vi "RobotSimulator.vi"() -> ()   [LabVIEW 2018]
uses:
  Robot-Project/Drive/Implementation/Drive Setpoints.ctl
  Robot-Project/Drive/Implementation/Drive Operations.ctl
  Controls/PurePursuit/RobotNeededPathData.ctl
  Robot-Project/Drive/DriveState.ctl
  <extravilib>/ChannelInstances/Lossy Stream-c(dbl,dbl,dbl,c(dbl,dbl))/Write With Abort.vi
  <extravilib>/ChannelInstances/Lossy Stream-c(dbl,dbl,dbl,c(dbl,dbl))/Read With Abort.vi
  <extravilib>/ChannelInstances/Lossy Stream-c(dbl,dbl,dbl,c(dbl,dbl))/Endpoint.vi
  <extravilib>/ChannelInstances/Lossy Stream-c(dbl,dbl,dbl,c(dbl,dbl))/EndpointRead.vi
  Robot-Project/Drive/Implementation/Drive Published Globals.vi
  <extravilib>/ChannelInstances/Lossy Stream-c(dbl,dbl,dbl,c(dbl,dbl))/Instantiate.vi
  <extravilib>/ChannelInstances/Lossy Stream-c(dbl,dbl,dbl,c(dbl,dbl))/)Channel.vi
  <resource>/ChannelSupport/_ChannelSupport/WaitIfNeeded.vi
  <vilib>/addons/control/pid/pid.llb/PID (DBL).vi
  Robot-Project/Configuration/Constants.vi
  <vilib>/addons/control/pid/NI_PID_pid.lvlib
  <extravilib>/ChannelInstances/Lossy Stream-c(dbl,dbl,dbl,c(dbl,dbl)).lvlib
panel:
  in  "Path":cluster{dbl, dbl}[](array[cluster])
  in  "Angle Addition":dbl(slide) scale=-180.0..180.0
  in  "Target":cluster{dbl, dbl}={200.0, 200.0}
  out "Current\nCmd":string="Started at  14:51:47.884\nDefault: Reserve,  L 0.0, R 0.0, D 0.000000"
  in  "Go":bool
  out "Loop Iterations":i32
  in  "Gains 2":T1={"Gains"={"FFV"=0.0055, "FFA"=0.0025, "Vel PID"={"P"=0.05, "I"=0.0, "D"=0.0}}, "Pos PID"={"P"=0.05, "I"=0.0, "D"=0.0}, "MinVoltage"=0.0, "Effective Trackwidth"=29.0, "Effective Trackwidth CCW"=29.0} {"Pos PID"."D" format="%.3f"; "Pos PID"."I" format="%.3f"; "Pos PID"."P" format="%.3f"; "Gains"."Vel PID"."D" format="%.3f"; "Gains"."Vel PID"."I" format="%.3f"; "Gains"."Vel PID"."P" format="%.3f"}
  out "Graph":cluster{cluster{"x":dbl, "y":dbl}[]}[](graph)=[{[]}, {[{"x"=19.5, "y"=127.60329985652797}, {"x"=31.499289530461766, "y"=127.73387843115106}]}, {[{"x"=0.0, "y"=0.0}]}, {[{"x"=19.5, "y"=127.60329985652797}, {"x"=19.5, "y"=127.60329985652797}, {"x"=19.5, "y"=127.60329985652797}, {"x"=19.5, "y"=127.60329985652797}, {"x"=19.5, "y"=127.60329985652797}, {"x"=19.5, "y"=127.60329985652797}, {"x"=19.5, "y"=127.60329985652797}, {"x"=19.5, "y"=127.60329985652797}, {"x"=19.5, "y"=127.60329985652797}, {"x"=19.5, "y"=127.60329985652797}, {"x"=19.5, "y"=127.60329985652797}, {"x"=19.5, "y"=127.60329985652797}, {"x"=19.5, "y"=127.60329985652797}, {"x"=19.5, "y"=127.60329985652797}, {"x"=19.5, "y"=127.60329985652797}, {"x"=19.5, "y"=127.60329985652797}, {"x"=19.5, "y"=127.60329985652797}, {"x"=19.5, "y"=127.60329985652797}, {"x"=19.5, "y"=127.60329985652797}, {"x"=19.5, "y"=127.60329985652797}, {"x"=19.5, "y"=127.60329985652797}, {"x"=19.5, "y"=127.60329985652797}, {"x"=19.5, "y"=127.60329985652797}, {"x"=19.5, "y"=127.60329985652797}, {"x"=19.5, "y"=127.60329985652797}, {"x"=19.5, "y"=127.60329985652797}, {"x"=19.5, "y"=127.60329985652797}, {"x"=19.5, "y"=127.60329985652797}, {"x"=19.5, "y"=127.60329985652797}, {"x"=19.5, "y"=127.60329985652797}, {"x"=19.5, "y"=127.60329985652797}]}, {[{"x"=inf, "y"=nan}, {"x"=inf, "y"=nan}, {"x"=inf, "y"=nan}, {"x"=inf, "y"=nan}, {"x"=inf, "y"=nan}, {"x"=inf, "y"=nan}, {"x"=inf, "y"=nan}, {"x"=inf, "y"=nan}, {"x"=nan, "y"=nan}, {"x"=nan, "y"=nan}, {"x"=nan, "y"=nan}, {"x"=nan, "y"=nan}, {"x"=nan, "y"=nan}, {"x"=nan, "y"=nan}, {"x"=nan, "y"=nan}, {"x"=nan, "y"=nan}, {"x"=nan, "y"=-inf}, {"x"=nan, "y"=-inf}, {"x"=nan, "y"=-inf}, {"x"=nan, "y"=-inf}, {"x"=nan, "y"=-inf}, {"x"=nan, "y"=-inf}, {"x"=nan, "y"=-inf}, {"x"=inf, "y"=-inf}, {"x"=inf, "y"=-inf}, {"x"=inf, "y"=-inf}, {"x"=inf, "y"=-inf}, {"x"=inf, "y"=-inf}, {"x"=inf, "y"=-inf}, {"x"=inf, "y"=-inf}, {"x"=inf, "y"=-inf}]}]
  out "Right Output":dbl
  out "Left Output":dbl
  in  "Config":T2={"Gear Reduction"=8.7, "Wheel Radius (m)"=0.076, "# Motors"=3, "coeff of friction"=0.1, "Mass (kg)"=55.0, "Motor"={"Ke (V)"=0.0183, "R (ohms)"=0.14, "KT (Nm/A)"=0.0183, "Tf (Nm)"=0.015}}
  in  "Position":dbl=3.0
  in  "Gains":T3={"FFV"=0.0059, "FFA"=0.0019, "Vel PID"={"P"=0.01, "I"=0.0, "D"=0.0}}
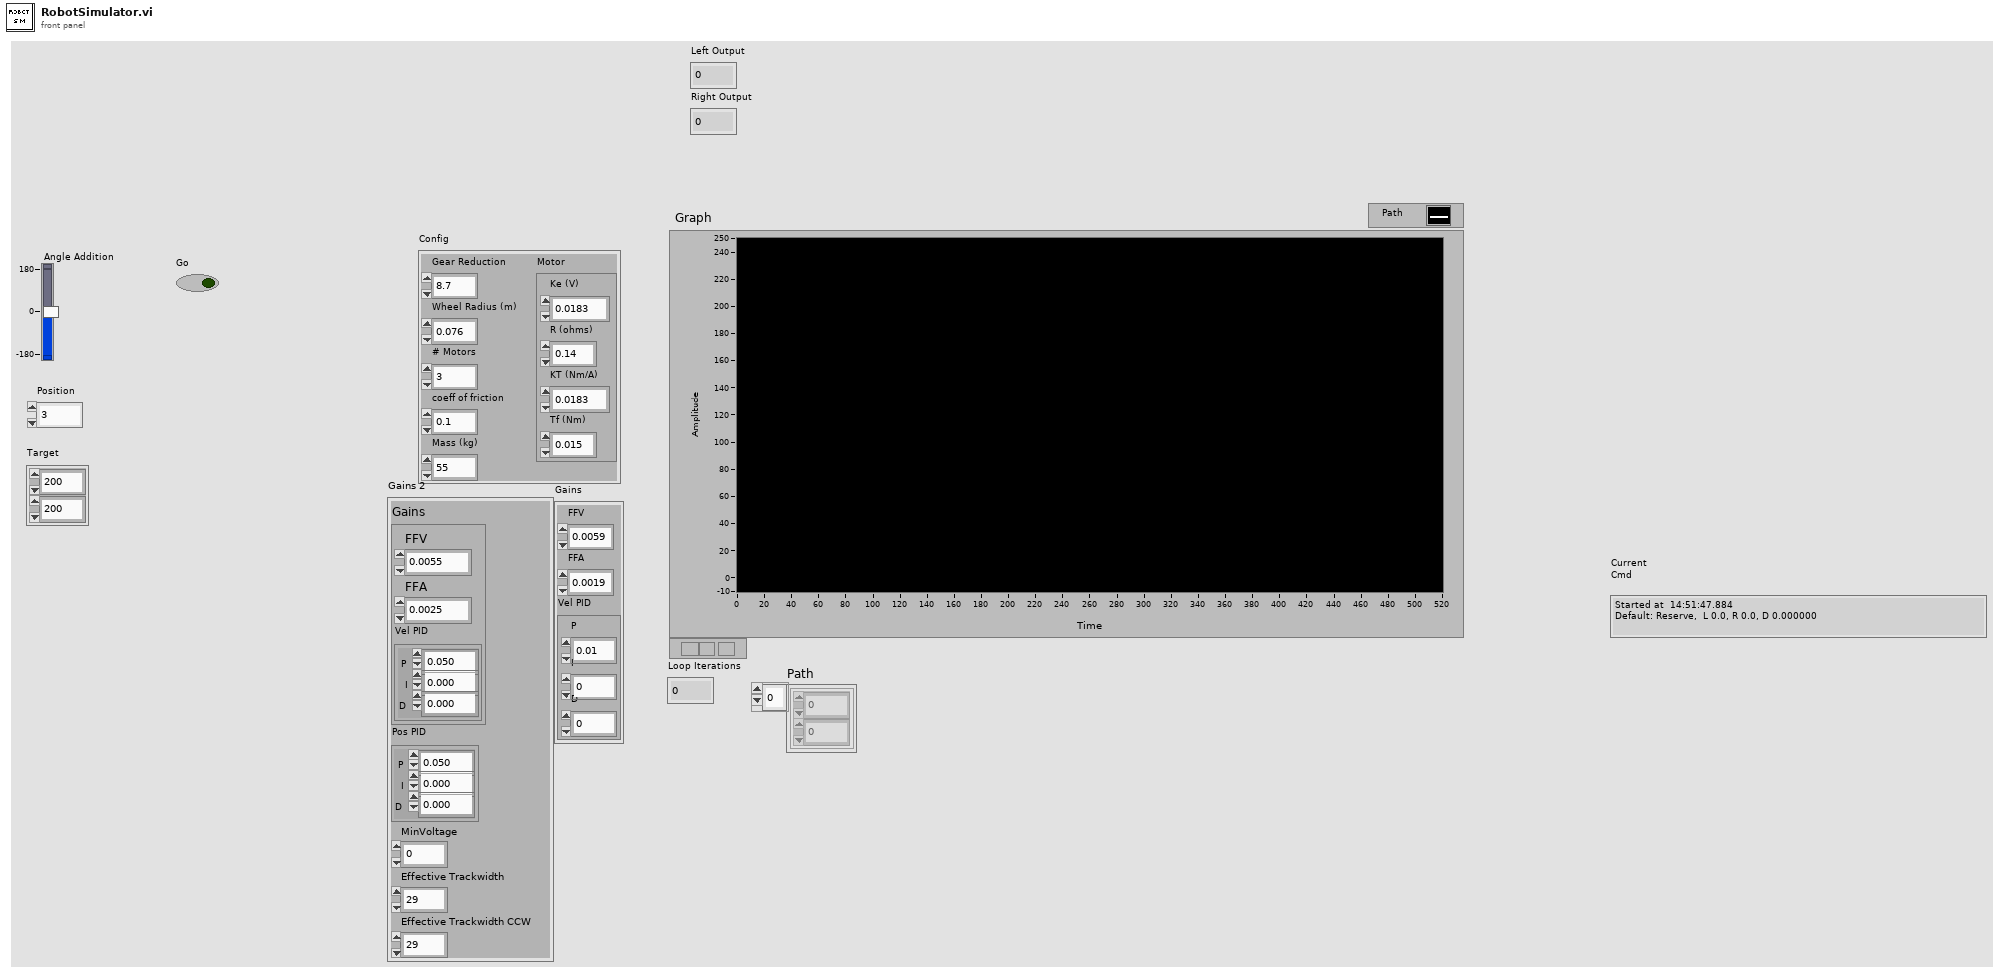
[diagram p1: front panel]
types:
  T1 = cluster{"Gains":cluster{"FFV":dbl, "FFA":dbl, "Vel PID":cluster{"P":dbl, "I":dbl, "D":dbl}}, "Pos PID":cluster{"P":dbl, "I":dbl, "D":dbl}, "MinVoltage":dbl, "Effective Trackwidth":dbl, "Effective Trackwidth CCW":dbl}
  T2 = cluster{"Gear Reduction":dbl, "Wheel Radius (m)":dbl, "# Motors":u32, "coeff of friction":dbl, "Mass (kg)":dbl, "Motor":cluster{"Ke (V)":dbl, "R (ohms)":dbl, "KT (Nm/A)":dbl, "Tf (Nm)":dbl}}
  T3 = cluster{"FFV":dbl, "FFA":dbl, "Vel PID":cluster{"P":dbl, "I":dbl, "D":dbl}}
  T4 = typedef "Drive Setpoints.ctl" = cluster{"Operation":T5, "Left Speed":dbl, "Right Speed":dbl, "Duration":dbl, "Speed":dbl, "Start Angle":dbl, "Target Angle":dbl, "Distance (inch)":dbl, "Start Point (inch)":dbl, "RobotNeededPathData":T6, "Start Point 2":dbl}
  T5 = typedef "Drive Operations.ctl" = enum16{"Reserve", "Read Current", "Immediate", "Drive for Time", "Drive for Distance", "Turn to Angle", "Drive Path"}
  T6 = typedef "RobotNeededPathData.ctl" = cluster{"Path":cluster{dbl, dbl}[], "MaxVel":dbl, "MaxAccel":dbl, "Backwards?":bool, "PointSpacing":dbl, "LookaheadDist":dbl, "Speed/Curve":dbl, "SlowDistanceAtEnd":dbl, "SlowSpeed":dbl, "MaxDeAccel":dbl}
  T7 = typedef "Command Status Info.ctl" = cluster{"Name":string, "Status":T8, "notifier out":T9}
  T8 = typedef "Completion Status.ctl" = enum16{"Successful", "Aborted", "Incomplete"}
  T9 = typedef "Completion Notifier.ctl" = refnum<notifier>
  T10 = cluster{"SubSystem Data":T4, cluster{"Start Time (ms)":u32, "Iterations":i32}, cluster{"Command Info":T7, "Description":string, "Default Command":T4, "queue out":refnum<queue>, "Subsystem Name":string}}
  T11 = typedef "DriveState.ctl" = enum16{"None", "Initial Turn", "Follow Path And Raise", "Align", "Score", "Backup And Lower"}
  T12 = cluster{"LeftVel":dbl, "RightVel":dbl, "Yaw":dbl, "Pos":cluster{"X":dbl, "Y":dbl}}
  T13 = typedef "Lossy Stream-c(dbl,dbl,dbl,c(dbl,dbl)).lvlib/)Channel.ctl" = refnum<queue>
  T14 = cluster{"proportional gain (Kc)":dbl, "integral time (Ti, min)":dbl, "derivative time (Td, min)":dbl}
  T15 = cluster{"Angle":dbl, "Angular vel":dbl, "Left Distance":dbl, "Left vel":dbl, "Right Distance":dbl, "Right vel":dbl}
  T16 = cluster{"LeftDistance":dbl, "RightDistance":dbl, "LeftVelocity":dbl, "RightVelocity":dbl, "Angle":dbl, "Location":cluster{dbl, dbl}}
  T17 = cluster{"dx/dt":dbl, "dx/dt":dbl, "Yaw":dbl, cluster{dbl, dbl}}
  T18 = cluster{"SubSystem Data":T4, cluster{"Start Time (ms)":u32, "Iterations":i32}, "Default Command Arguments":cluster{"Command Info":T7, "Description":string, "Default Command":T4, "queue out":refnum<queue>, "Subsystem Name":string}}
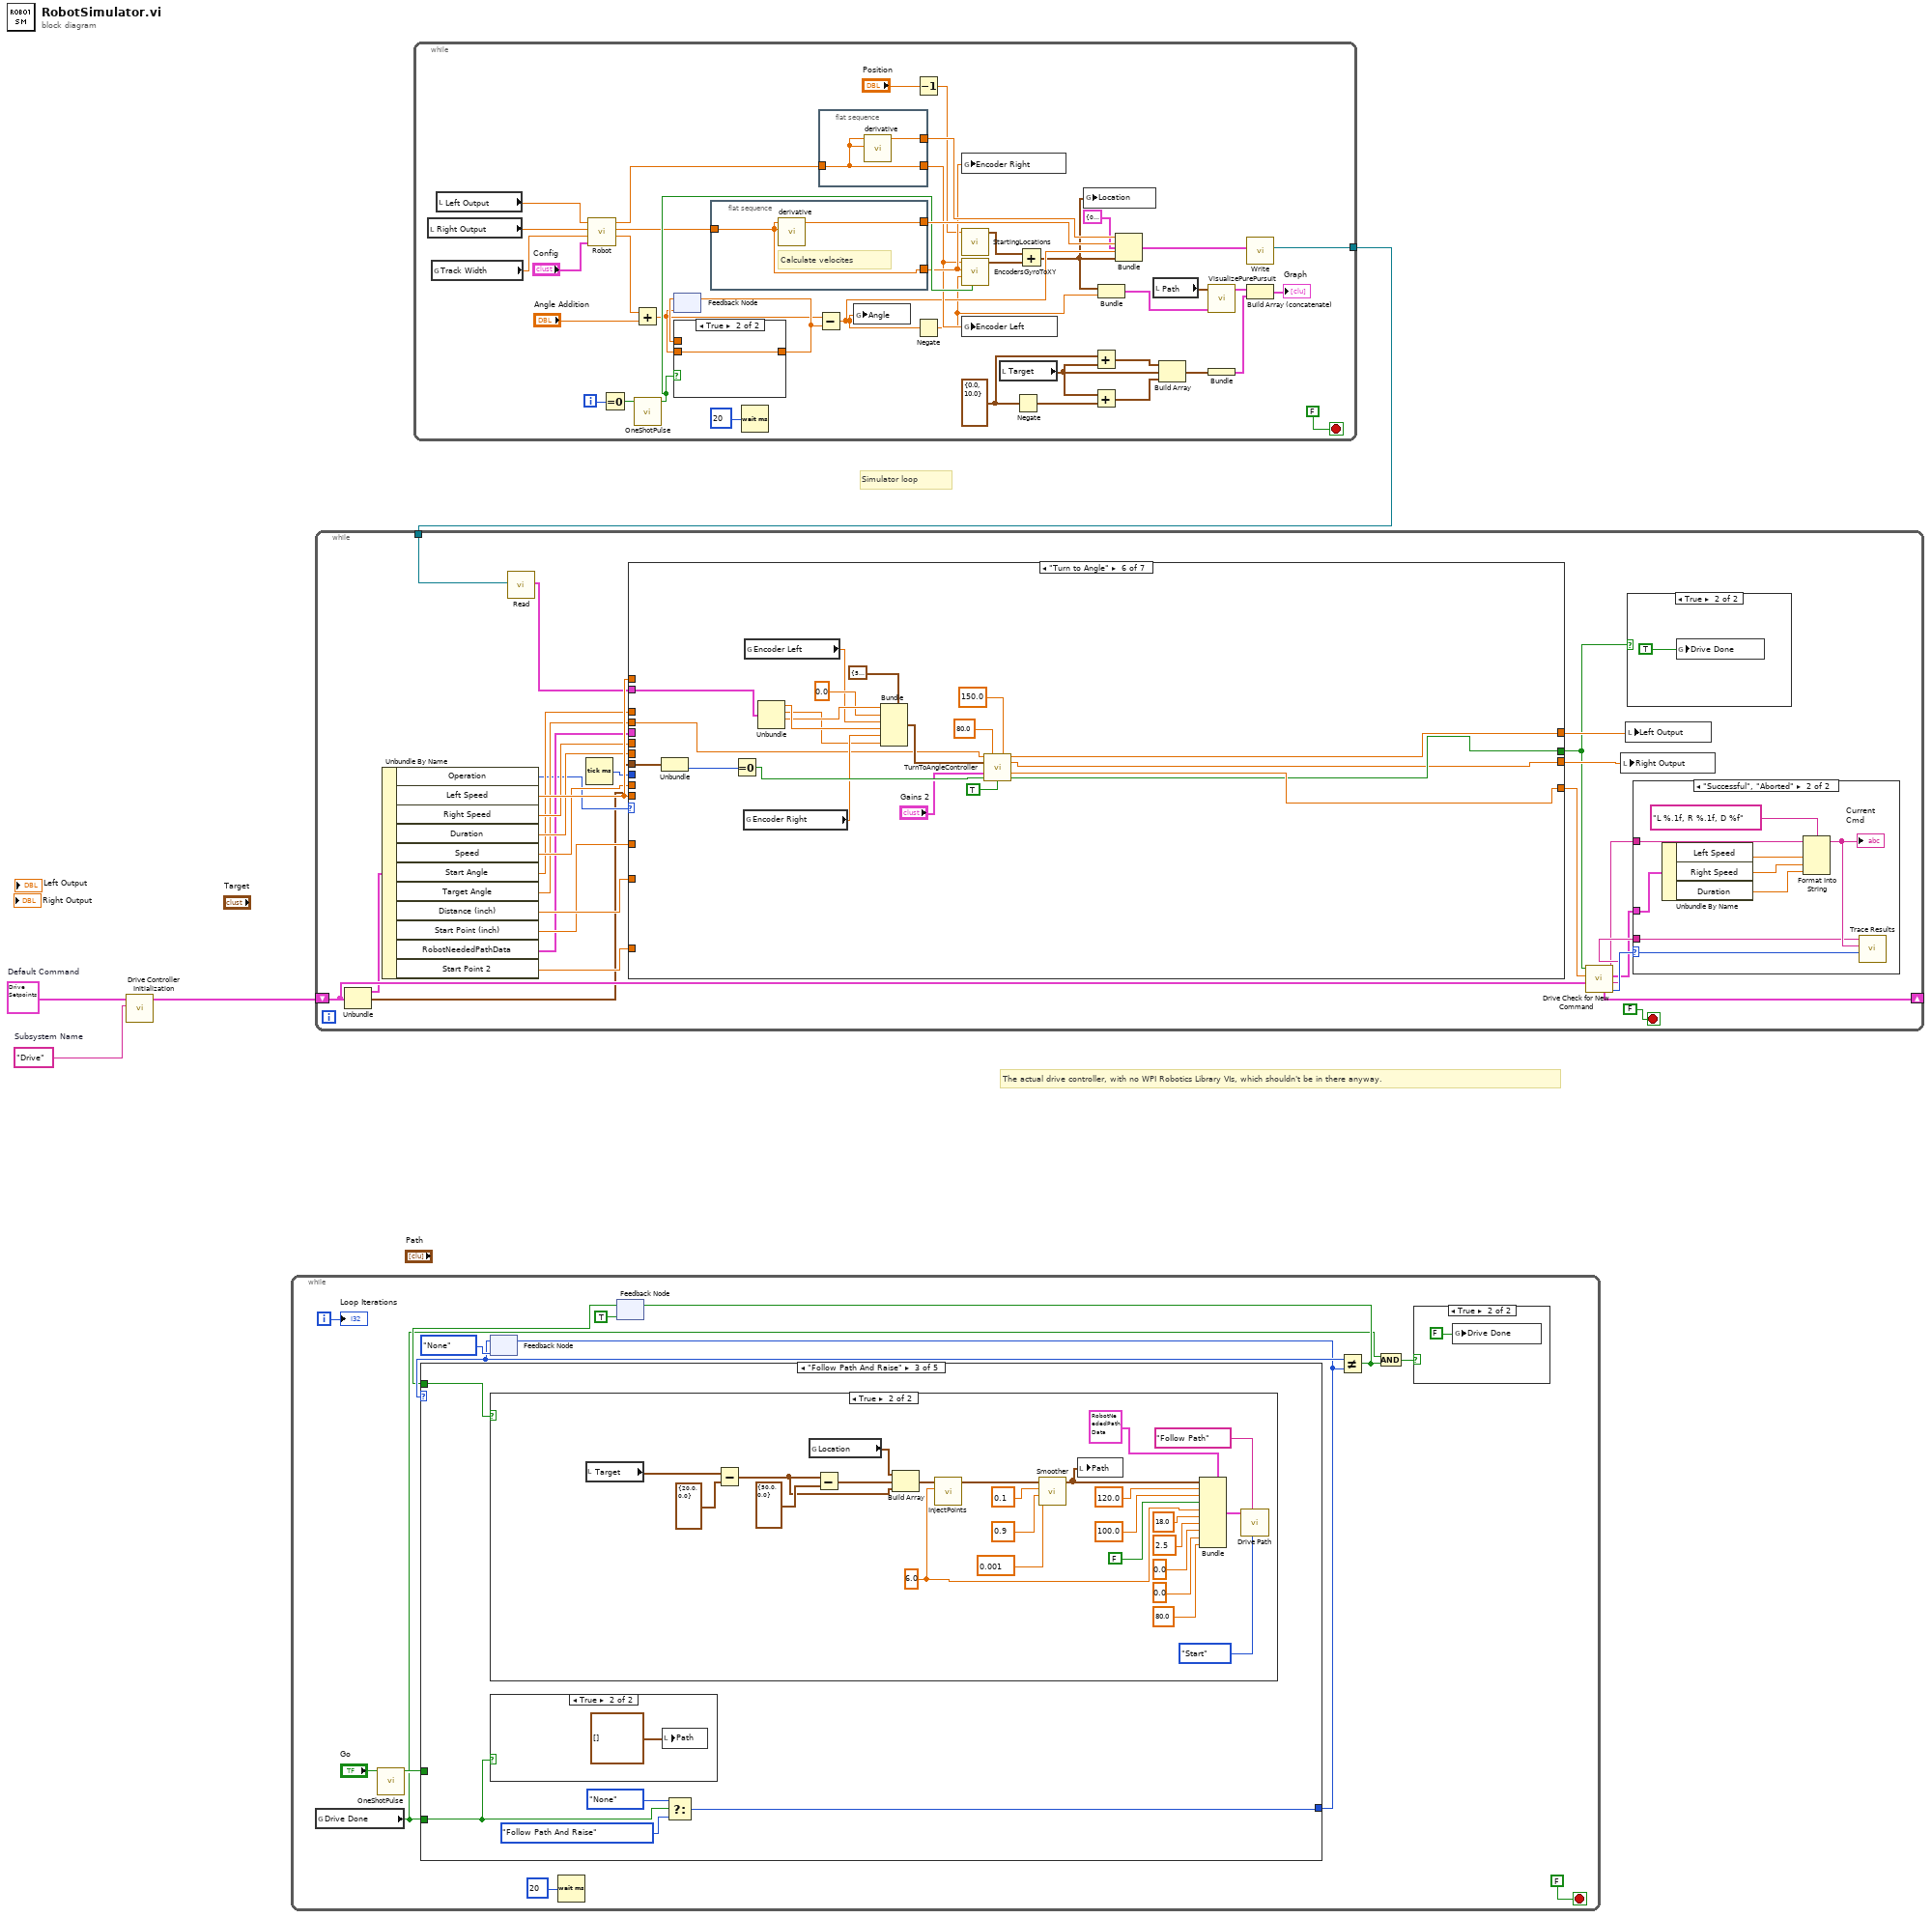
[diagram p0: block diagram]
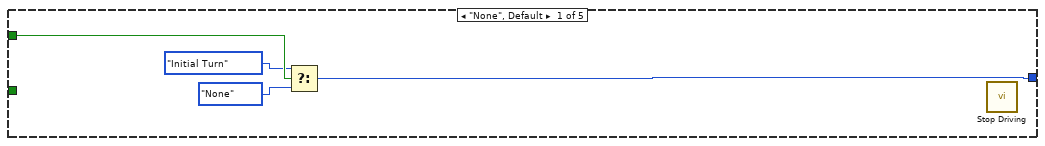
[diagram p3: hidden frame]
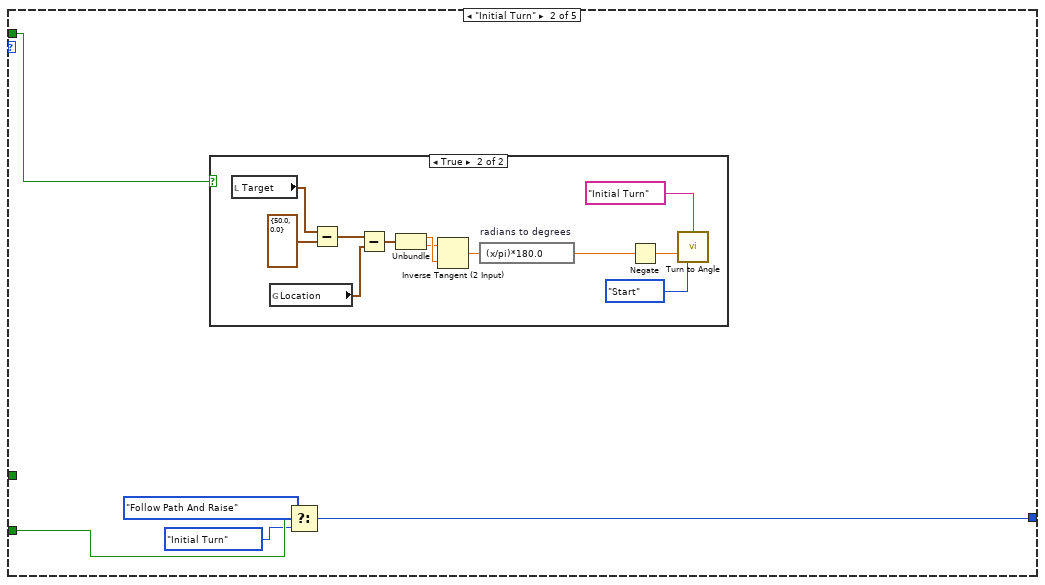
[diagram p4: hidden frame]
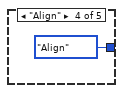
[diagram p8: hidden frame]
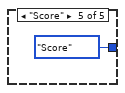
[diagram p9: hidden frame]
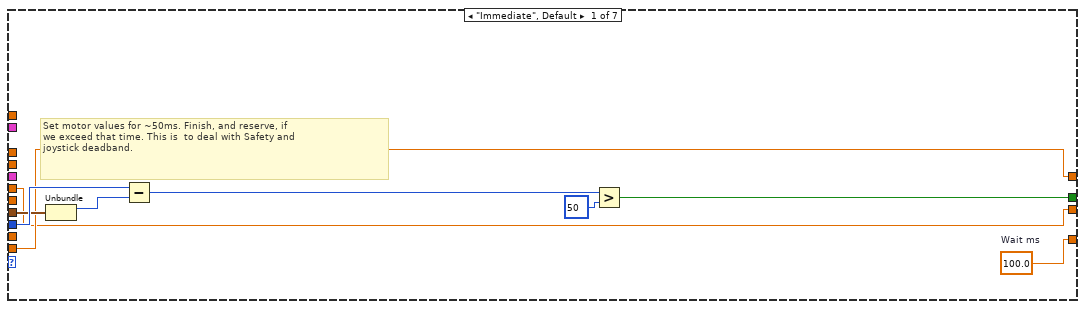
[diagram p13: hidden frame]
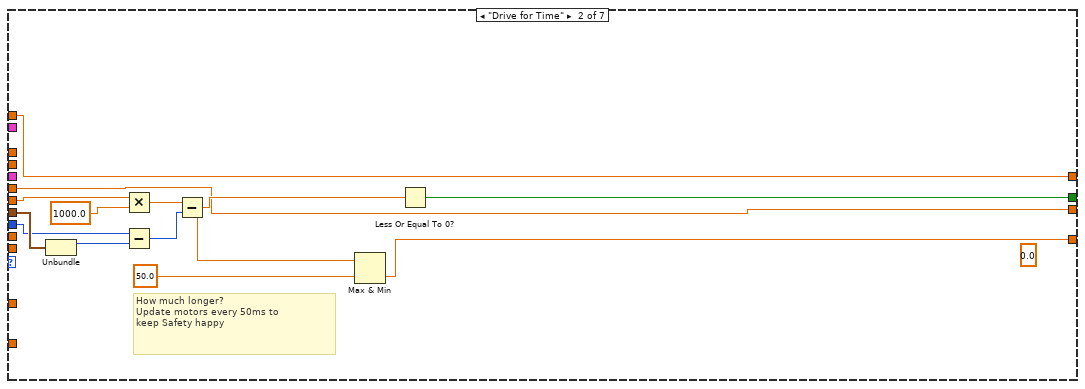
[diagram p14: hidden frame]
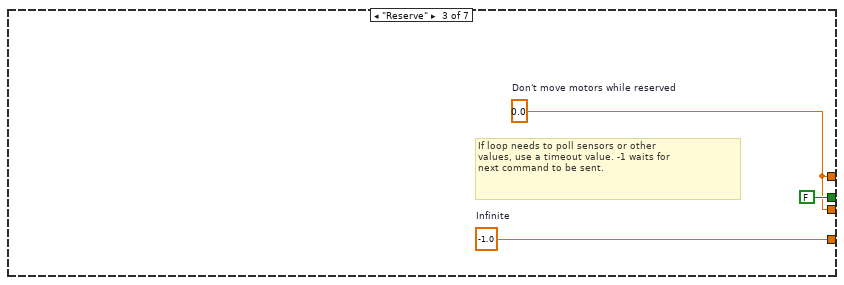
[diagram p15: hidden frame]
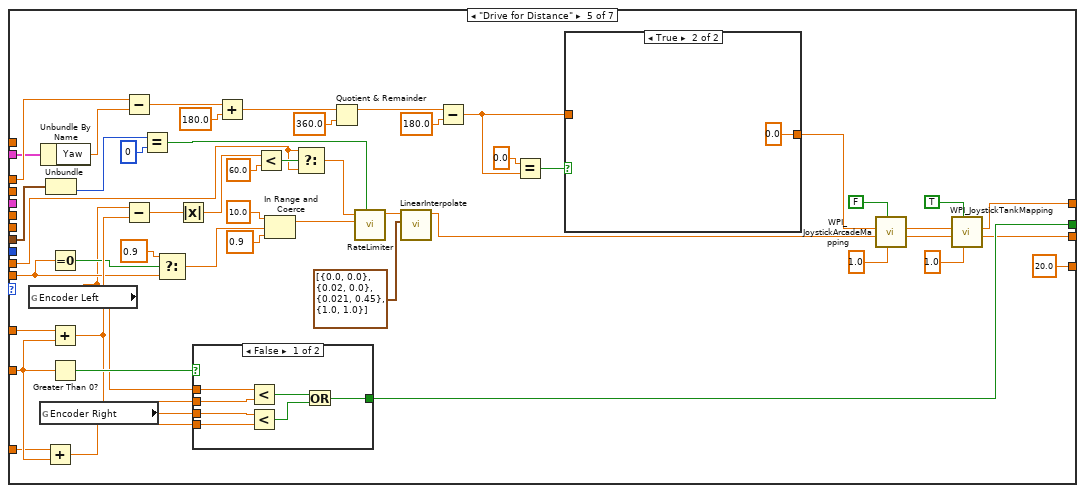
[diagram p17: hidden frame]
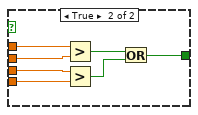
[diagram p18: hidden frame]
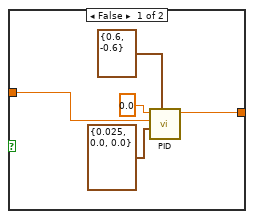
[diagram p19: hidden frame]
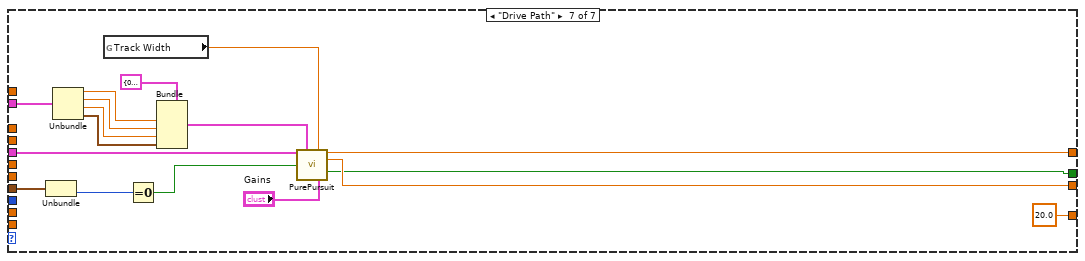
[diagram p20: hidden frame]
diagram:
  w3 = T4 {"Operation"=enum."Reserve", "Left Speed"=0.0, "Right Speed"=0.0, "Duration"=0.0, "Speed"=0.0, "Start Angle"=0.0, "Target Angle"=0.0, "Distance (inch)"=0.0, "Start Point (inch)"=0.0, "RobotNeededPathData"={"Path"=[], "MaxVel"=0.0, "MaxAccel"=0.0, "Backwards?"=FALSE, "PointSpacing"=0.0, "LookaheadDist"=0.0, "Speed/Curve"=1.8, "SlowDistanceAtEnd"=12.0, "SlowSpeed"=15.0, "MaxDeAccel"=0.0}, "Start Point 2"=0.0}  # Default Command
  w4 = "Drive"  # Subsystem Name
  # "Simulator loop"
  # "The actual drive controller, with no WPI Robotics Library VIs, which shouldn't be in there anyway."
  n1 = call "Drive Controller Initialization.vi"("Subsystem Name"=w4, "Default Command"=w3) -> ("Current Command"=w2:T10)  [unwired: 9 in]
  n2 = while {
    i -> [w15]
    stop <- FALSE stop-if-true
    n3 = global read "Drive Published Globals.vi" "Drive Done"() -> (w5:bool)
    n4 = call "OneShotPulse.vi"("Input"="Go") -> ("Output"=w12:bool)  [unwired: 10 in]
    n5 = feedback #1(DriveState."None" ("State")) -> (w11:T11)
    n6 = Wait (ms)(milliseconds to wait=u32 20) -> ()  [unwired: 1 out]
    n7 = feedback #2(TRUE) -> (w8:bool)
    n8 = case shown="\"Follow Path And Raise\"" w11 {
      tunnel: w12 -> [w22 _ _ _ _]
      tunnel: [w20 w25 w43 DriveState."Align" ("f") DriveState."Score" ("f")] -> w10
      tunnel: w8 -> [_ w27 w44 _ _]
      tunnel: w5 -> [_ w26 w40 _ _]
      frame "None", Default {
        n9 = Select(t=DriveState."Initial Turn", s=w22, f=DriveState."None" ("State")) -> (s? t:f=w20:T11)
        n10 = call "Stop Driving.vi"() -> ()  [unwired: 11 in, 1 out]
      }
      frame "Initial Turn" {
        n11 = case shown="True" w27 {
          frame False {
          }
          frame True {
            n12 = local read "Target"() -> (w30:cluster{dbl, dbl})
            n13 = global read "Drive Published Globals.vi" "Location"() -> (w37:cluster{dbl, dbl})
            n14 = Subtract(x=w30, y=cluster{dbl, dbl} {50.0, 0.0}) -> (x-y=w28:cluster{dbl, dbl})
            n15 = Subtract(x=w28, y=w37) -> (x-y=w36:cluster{dbl, dbl})
            n16 = Unbundle(w36) -> (w35:dbl, w34:dbl)
            n17 = Inverse Tangent (2 Input)(1:w35, 2:w34) -> (0:w33:dbl)
            n18 = expression code="(x/pi)*180.0" "radians to degrees"(w33) -> (w32:dbl)
            n19 = Negate(x=w32) -> (-x=w31:dbl)
            n20 = call "Turn to Angle.vi"("Description"="Initial Turn", "Target Angle"=w31, "Synchronication"=enum16{"Start", "Wait"}."Start") -> ()  [unwired: 12 in, 1 out]
          }
        }
        n21 = Select(t=DriveState."Follow Path And Raise" ("State"), s=w26, f=DriveState."Initial Turn" ("State")) -> (s? t:f=w25:T11)
      }
      frame "Follow Path And Raise" {
        n22 = case shown="True" w44 {
          frame False {
          }
          frame True {
            w55 = 6.0 ("Distance")
            n23 = local read "Target"() -> (w69:cluster{dbl, dbl})
            n24 = Subtract(x=w69, y=cluster{dbl, dbl} {20.0, 0.0}) -> (x-y=w64:cluster{dbl, dbl})
            n25 = global read "Drive Published Globals.vi" "Location"() -> (w66:cluster{dbl, dbl})
            n26 = Subtract(x=w64, y=cluster{dbl, dbl} {50.0, 0.0}) -> (x-y=w65:cluster{dbl, dbl})
            n27 = Build Array(w66, w65, w64) -> (w60:cluster{dbl, dbl}[])
            n28 = call "InjectPoints.vi"("Spacing"=w55, "Path"=w60) -> ("Path out"=w47:cluster{dbl, dbl}[])  [unwired: 9 in]
            n29 = call "Smoother.vi"("tolerance"=0.001, "B"=0.9, "A"=0.1, "Path"=w47) -> ("SmoothPath"=w46:cluster{dbl, dbl}[])  [unwired: 7 in]
            n30 = local write "Path"(w46) -> ()
            n31 = Bundle(cluster=T6 {"Path"=[], "MaxVel"=0.0, "MaxAccel"=0.0, "Backwards?"=FALSE, "PointSpacing"=0.0, "LookaheadDist"=0.0, "Speed/Curve"=1.8, "SlowDistanceAtEnd"=12.0, "SlowSpeed"=15.0, "MaxDeAccel"=0.0} ("Path"), "Path"=w46, "MaxVel"=120.0, "MaxAccel"=100.0, "Backwards?"=FALSE, "PointSpacing"=w55, "LookaheadDist"=18.0, "Speed/Curve"=2.5, "SlowDistanceAtEnd"=0.0, "SlowSpeed"=0.0, "MaxDeAccel"=80.0) -> (w49:T6)
            n32 = call "Drive Path.vi"("Synchronication"=enum16{"Start", "Wait"}."Start", "Description"="Follow Path", "Path"=w49) -> ()  [unwired: 8 in, 1 out]
          }
        }
        n33 = case shown="True" w40 {
          frame False {
          }
          frame True {
            n34 = local write "Path"(cluster{dbl, dbl}[] [] ("Path")) -> ()
          }
        }
        n35 = Select(t=DriveState."None" ("State"), s=w40, f=DriveState."Follow Path And Raise") -> (s? t:f=w43:T11)
      }
      frame "Align" {
      }
      frame "Score" {
      }
    }
    n36 = feedback-in #1(w10) -> ()
    n37 = Not Equal?(x=w11, y=w10) -> (x != y?=w7:bool)
    n38 = feedback-in #2(w7) -> ()
    n39 = And(x=w5, y=w7) -> (x .and. y?=w6:bool)
    n40 = case shown="True" w6 {
      frame False {
      }
      frame True {
        n41 = global write "Drive Published Globals.vi" "Drive Done"(FALSE ("Command Done")) -> ()
      }
    }
    "Loop Iterations" <- w15
  }
  n42 = while {
    tunnel: [w100] -> w1
    i -> [w99]
    stop <- FALSE stop-if-true
    w80 = cluster{dbl, dbl} {0.0, 10.0} ("x")
    n43 = local read "Right Output"() -> (w94:dbl)
    n44 = global read "Constants.vi" "Track Width"() -> (w95:dbl)
    n45 = local read "Left Output"() -> (w93:dbl)
    n46 = call "Robot.vi"("Config"="Config", "WheelBase"=w95, "Right Value"=w94, "Left Value"=w93) -> ("Angle"=w83:dbl, "Right Distance"=w88:dbl, "Left Distance"=w89:dbl)  [unwired: 5 in]
    n47 = Equal To 0?(x=w99) -> (x = 0?=w98:bool)
    n48 = Add(x=w83, y="Angle Addition") -> (x+y=w81:dbl)
    n49 = call "OneShotPulse.vi"("Input"=w98) -> ("Output"=w107:bool)  [unwired: 10 in]
    n50 = feedback #3(w81) -> (w108:dbl)
    n51 = case shown="True" w107 {
      tunnel: w81 -> [_ w117]
      tunnel: [w116 w117] -> w109
      tunnel: w108 -> [w116 _]
      frame False {
      }
      frame True {
      }
    }
    n52 = feedback-in #3(w109) -> ()
    n53 = flat-sequence {
      tunnel: [w119] -> w111
      tunnel: [w118] -> w105
      tunnel: w88 -> [w118]
      frame #0 {
        # "Calculate velocites"
        n54 = call "derivative.vi"("Starting value"=w118, "x"=w118) -> ("dx/dt"=w119:dbl)  [unwired: 9 in]
      }
    }
    n55 = Wait (ms)(milliseconds to wait=u32 20) -> ()  [unwired: 1 out]
    n56 = Subtract(x=w81, y=w109) -> (x-y=w103:dbl)
    n57 = flat-sequence {
      tunnel: [w115] -> w106
      tunnel: [w114] -> w104
      tunnel: w89 -> [w114]
      frame #0 {
        n58 = call "derivative.vi"("Starting value"=w114, "x"=w114) -> ("dx/dt"=w115:dbl)  [unwired: 9 in]
      }
    }
    n59 = global write "Drive Published Globals.vi" "Angle"(w103) -> ()
    n60 = Decrement(x="Position") -> (x-1=w74:dbl)
    n61 = Negate(x=w103) -> (-x=w90:dbl)
    n62 = global write "Drive Published Globals.vi" "Encoder Right"(w105) -> ()
    n63 = call "StartingLocations.vi"("Index"=w74) -> ("Location"=w73:cluster{dbl, dbl})  [unwired: 10 in]
    n64 = call "EncodersGyroToXY.vi"("Reset"=w107, "Angle (degrees)"=w90, "Right Distance"=w105, "Left Distance"=w104) -> ("Location"=w110:cluster{dbl, dbl})  [unwired: 7 in]
    n65 = global write "Drive Published Globals.vi" "Encoder Left"(w104) -> ()
    n66 = local read "Target"() -> (w77:cluster{dbl, dbl})
    n67 = Negate(x=w80) -> (-x=w79:cluster{dbl, dbl})
    n68 = Add(x=w73, y=w110) -> (x+y=w92:cluster{dbl, dbl})
    n69 = global write "Drive Published Globals.vi" "Location"(w92) -> ()
    n70 = Add(x=w80, y=w77) -> (x+y=w78:cluster{dbl, dbl})
    n71 = Add(x=w77, y=w79) -> (x+y=w76:cluster{dbl, dbl})
    n72 = Bundle(w92, w90) -> (w91:cluster{cluster{dbl, dbl}, dbl})  [unwired: 1 in]
    n73 = Bundle(cluster=T12 {"LeftVel"=0.0, "RightVel"=0.0, "Yaw"=0.0, "Pos"={"X"=0.0, "Y"=0.0}} ("Robot"), "LeftVel"=w106, "RightVel"=w111, "Yaw"=w103, "Pos"=w92) -> (w101:T12)
    n74 = local read "Path"() -> (w75:cluster{dbl, dbl}[])
    n75 = Build Array(w78, w77, w76) -> (w87:cluster{dbl, dbl}[])
    n76 = call "VisualizePurePursuit.vi"("Robot"=w91, "Path"=w75) -> ("Graph"=w86:cluster{cluster{"x":dbl, "y":dbl}[]}[])  [unwired: 9 in]
    n77 = Bundle(w87) -> (w84:cluster{cluster{dbl, dbl}[]})  [unwired: 1 in]
    n78 = call <extravilib>:"Write.vi"("element"=w101) -> ("channel"=w100:T13)  [unwired: 8 in, 2 out]
    n79 = Build Array (concatenate)(w86, w84) -> (→"Graph":cluster{cluster{"x":dbl, "y":dbl}[]}[])
  }
  n80 = while {
    shift-right: [w146] -> _
    shift-left: w2 -> [w144]
    tunnel: w1 -> [w128]
    stop <- FALSE stop-if-true
    n81 = Unbundle(w144) -> ("SubSystem Data"=w130:T4, w129:cluster{"Start Time (ms)":u32, "Iterations":i32})  [unwired: 1 out]
    n82 = Unbundle By Name(w130) -> ("Operation"=w133:T5, "Left Speed"=w143:dbl, "Right Speed"=w142:dbl, "Duration"=w141:dbl, "Speed"=w140:dbl, "Start Angle"=w139:dbl, "Target Angle"=w138:dbl, "Distance (inch)"=w137:dbl, "Start Point (inch)"=w136:dbl, "RobotNeededPathData"=w135:T6, "Start Point 2"=w134:dbl)
    n83 = call <extravilib>:"Read.vi"("channel"=w128) -> ("element"=w127:T17)  [unwired: 5 in, 5 out]
    n84 = Tick Count (ms)() -> (millisecond timer value=w132:u32)
    n85 = case shown="\"Turn to Angle\"" w133 {
      tunnel: [w165 w169 w181 _ 20.0 ("Infinite") w270 20.0 ("Infinite")] -> w131
      tunnel: [w160 w173 FALSE ("ignore previous (F)") _ w223 w269 w287] -> w120
      tunnel: w129 -> [w159 w175 _ _ w206 w273 w277]
      tunnel: w132 -> [w161 w172 _ _ _ _ _]
      tunnel: [w158 w167 w179 _ w211 w268 w289] -> w121
      tunnel: [w157 w166 w179 _ w212 w267 w288] -> w126
      tunnel: w140 -> [_ _ _ _ w196 _ _]
      tunnel: w137 -> [_ _ _ _ w195 _ _]
      tunnel: w141 -> [_ w168 _ _ _ _ _]
      tunnel: w143 -> [w158 _ _ _ w190 _ _]
      tunnel: w142 -> [w157 w166 _ _ _ _ _]
      tunnel: w139 -> [_ _ _ _ w218 _ _]
      tunnel: w138 -> [_ _ _ _ _ w256 _]
      tunnel: w136 -> [_ _ _ _ w217 _ _]
      tunnel: w143 -> [_ w167 _ _ _ _ _]
      tunnel: w135 -> [_ _ _ _ _ _ w290]
      tunnel: w127 -> [_ _ _ _ w185 w264 w281]
      tunnel: w134 -> [_ _ _ _ w194 _ _]
      frame "Immediate", Default {
        w165 = 100.0  # Wait ms
        # "Set motor values for ~50ms. Finish, and reserve, if\nwe exceed that time. This is  to deal with Safety and\njoystick deadband."
        n86 = Unbundle(w159) -> ("Start Time (ms)"=w162:u32)  [unwired: 1 out]
        n87 = Subtract(x=w161, y=w162) -> (x-y=w163:u32)
        n88 = Greater?(x=w163, y=u8 50 ("Left Motor")) -> (0:w160:bool)
      }
      frame "Drive for Time" {
        (unwired) 0.0 ("output")
        # "How much longer?\nUpdate motors every 50ms to\nkeep Safety happy"
        n89 = Unbundle(w175) -> ("Start Time (ms)"=w174:u32)  [unwired: 1 out]
        n90 = Multiply(x=w168, y=1000.0) -> (x*y=w177:dbl)
        n91 = Subtract(x=w172, y=w174) -> (x-y=w178:u32)
        n92 = Subtract(x=w177, y=w178) -> (x-y=w171:dbl)
        n93 = Max & Min(x=w171, y=50.0) -> (min(x,y)=w169:dbl)  [unwired: 1 out]
        n94 = Less Or Equal To 0?(x=w171) -> (x <= 0?=w173:bool)
      }
      frame "Reserve" {
        w179 = 0.0  # Don't move motors while reserved
        w181 = -1.0  # Infinite
        # "If loop needs to poll sensors or other\nvalues, use a timeout value. -1 waits for\nnext command to be sent."
      }
      frame "Read Current" {
      }
      frame "Drive for Distance" {
        n95 = global read "Drive Published Globals.vi" "Encoder Left"() -> (w183:dbl)
        n96 = global read "Drive Published Globals.vi" "Encoder Right"() -> (w182:dbl)
        n97 = Unbundle By Name(w185) -> ("Yaw"=w184:dbl)
        n98 = Add(x=w194, y=w195) -> (x+y=w193:dbl)
        n99 = Unbundle(w206) -> ("Iterations"=w205:i32)  [unwired: 1 out]
        n100 = Equal To 0?(x=w190) -> (x = 0?=w192:bool)
        n101 = Add(x=w217, y=w195) -> (x+y=w202:dbl)
        n102 = Greater Than 0?(x=w195) -> (x > 0?=w216:bool)
        n103 = Subtract(x=w218, y=w184) -> (x-y=w225:dbl)
        n104 = Subtract(x=w183, y=w202) -> (x-y=w201:dbl)
        n105 = Equal?(x=w205, y=0) -> (x = y?=w203:bool)
        n106 = Select(t=0.9, s=w192, f=w190) -> (s? t:f=w189:dbl)
        n107 = Absolute Value(x=w201) -> (abs(x)=w200:dbl)
        n108 = case shown="False" w216 {
          tunnel: w183 -> [w238 w246]
          tunnel: w202 -> [w239 w245]
          tunnel: [w236 w240] -> w223
          tunnel: w193 -> [w234 w244]
          tunnel: w182 -> [w235 w243]
          frame False {
            n109 = Less?(x=w238, y=w239) -> (x < y?=w237:bool)
            n110 = Less?(x=w235, y=w234) -> (x < y?=w233:bool)
            n111 = Or(x=w237, y=w233) -> (x .or. y?=w236:bool)
          }
          frame True {
            n112 = Greater?(x=w246, y=w245) -> (0:w242:bool)
            n113 = Greater?(x=w243, y=w244) -> (0:w241:bool)
            n114 = Or(x=w242, y=w241) -> (x .or. y?=w240:bool)
          }
        }
        n115 = Add(x=w225, y=180.0) -> (x+y=w229:dbl)
        n116 = Less?(x=w200, y=60.0) -> (x < y?=w198:bool)
        n117 = In Range and Coerce(upper limit=10.0, x=w189, lower limit=0.9) -> (coerced(x)=w186:dbl)  [unwired: 1 out]
        n118 = Select(t=w196, s=w198, f=w196) -> (s? t:f=w197:dbl)
        n119 = Quotient & Remainder(x=w229, y=360.0) -> (x-y*floor(x/y)=w227:dbl)  [unwired: 1 out]
        n120 = call "RateLimiter.vi"("Reset"=w203, "Max dx/dt"=w186, "Input"=w197) -> ("Output"=w214:dbl)  [unwired: 8 in]
        n121 = call "LinearInterpolate.vi"("Points"=cluster{"X":dbl, "Y":dbl}[] [{"X"=0.0, "Y"=0.0}, {"X"=0.02, "Y"=0.0}, {"X"=0.021, "Y"=0.45}, {"X"=1.0, "Y"=1.0}], "Value"=w214) -> ("Output"=w215:dbl)  [unwired: 9 in]
        n122 = Subtract(x=w227, y=180.0) -> (x-y=w224:dbl)
        n123 = Equal?(x=0.0, y=w224) -> (x = y?=w232:bool)
        n124 = case shown="True" w232 {
          tunnel: [w247 0.0] -> w219
          tunnel: w224 -> [w248 _]
          frame False {
            n125 = call-poly <vilib>:"PID.vi"("output range"=cluster{"output high":dbl, "output low":dbl} {"output high"=0.6, "output low"=-0.6}, "PID gains"=T14 {"proportional gain (Kc)"=0.025, "integral time (Ti, min)"=0.0, "derivative time (Td, min)"=0.0}, "process variable"=w248, "setpoint"=0.0) -> ("output"=w247:dbl)  [unwired: 6 in, 1 out]
          }
          frame True {
          }
        }
        n126 = call <vilib>:"WPI_JoystickArcadeMapping.vi"("Max Output"=1.0, "Square Inputs"=FALSE, "Y axis value"=w215, "X axis value"=w219) -> ("Right Motor Value"=w210:dbl, "Left Motor Value"=w209:dbl)  [unwired: 6 in]
        n127 = call <vilib>:"WPI_JoystickTankMapping.vi"("Max Output"=1.0, "Square Inputs"=TRUE, "Right axis value"=w210, "Left axis value"=w209) -> ("Right Motor Value"=w212:dbl, "Left Motor Value"=w211:dbl)  [unwired: 6 in]
      }
      frame "Turn to Angle" {
        n128 = Unbundle(w273) -> ("Iterations"=w272:i32)  [unwired: 1 out]
        n129 = Equal To 0?(x=w272) -> (x = 0?=w271:bool)
        n130 = global read "Drive Published Globals.vi" "Encoder Right"() -> (w259:dbl)
        n131 = global read "Drive Published Globals.vi" "Encoder Left"() -> (w260:dbl)
        n132 = Unbundle(w264) -> ("dx/dt"=w263:dbl, "dx/dt"=w254:dbl, "Yaw"=w262:dbl)  [unwired: 1 out]
        n133 = Bundle(cluster=T15 {"Angle"=548.1299999999924, "Angular vel"=0.49263510517714687, "Left Distance"=26.0882735, "Left vel"=0.0, "Right Distance"=-234.57467250000002, "Right vel"=0.0} ("Robot"), "Angle"=w262, "Angular vel"=0.0, "Left Distance"=w260, "Left vel"=w263, "Right Distance"=w259, "Right vel"=w254) -> (w266:T15)
        n134 = call "TurnToAngleController.vi"("TargetAngle"=w256, "MaxVel"=80.0, "MaxAccel"=150.0, "Robot"=w266, "Gains"="Gains 2", "Reset"=w271, "GoSmallestDistance"=TRUE) -> ("LeftPower"=w268:dbl, "RightPower"=w267:dbl, "Delay"=w270:dbl, "Done"=w269:bool)  [unwired: 2 in, 3 out]
      }
      frame "Drive Path" {
        n135 = Unbundle(w277) -> ("Iterations"=w278:i32)  [unwired: 1 out]
        n136 = Unbundle(w281) -> ("dx/dt"=w285:dbl, "dx/dt"=w284:dbl, "Yaw"=w283:dbl, w282:cluster{dbl, dbl})
        n137 = global read "Constants.vi" "Track Width"() -> (w276:dbl)
        n138 = Equal To 0?(x=w278) -> (x = 0?=w279:bool)
        n139 = Bundle(cluster=T16 {"LeftDistance"=0.0, "RightDistance"=0.0, "LeftVelocity"=0.0, "RightVelocity"=0.0, "Angle"=0.0, "Location"={0.0, 0.0}} ("SensorData"), "LeftVelocity"=w285, "RightVelocity"=w284, "Angle"=w283, "Location"=w282) -> (w286:T16)  [unwired: 2 in]
        n140 = call "PurePursuit.vi"("RobotNeededPathData"=w290, "SensorData"=w286, "Trackwidth"=w276, "Reset"=w279, "Gains"="Gains") -> ("LeftValue"=w289:dbl, "RightValue"=w288:dbl, "Done"=w287:bool)  [unwired: 6 in, 2 out]
      }
    }
    n141 = call "Drive Check for New Command.vi"("input cluster"=w144, "Wait time (ms)"=w131, "Finished?"=w120) -> ("Completion"=w125:T8, "Subsystem Name"=w124:string, "Current Command"=w123:T4, "Initial Trace String"=w122:string, "Next Command"=w146:T18)  [unwired: 4 in]
    n142 = local write "Right Output"(w126) -> ()
    n143 = local write "Left Output"(w121) -> ()
    n144 = case shown="True" w120 {
      frame False {
      }
      frame True {
        n145 = global write "Drive Published Globals.vi" "Drive Done"(TRUE ("Command Done")) -> ()
      }
    }
    n146 = case shown="\"Successful\", \"Aborted\"" w125 {
      selector: w125 -> [_ w156]
      tunnel: w122 -> [_ w151]
      tunnel: w123 -> [_ w152]
      tunnel: w124 -> [_ w148]
      frame "Incomplete", Default {
        # "Continuing current command"
      }
      frame "Successful", "Aborted" {
        # "Report and setup for next command"
        n147 = Unbundle By Name(w152) -> ("Left Speed"=w154:dbl, "Right Speed"=w155:dbl, "Duration"=w149:dbl)
        n148 = Format Into String(format string="L %.1f, R %.1f, D %f", initial string=w151, w154, w155, w149) -> (resulting string=w150:string)  [unwired: 1 in, 1 out]
        "Current\nCmd" <- w150
        n149 = call <vilib>:"Trace Results.vi"("Status of previous command"=w156, "Description"=w150, "Subsystem"=w148) -> ()  [unwired: 9 in]
      }
    }
  }
